vi "PH_PPMA_PowerUnit.panel.vi"() -> ()   [LabVIEW 2014, in "PH_PPMA_PowerUnit.lvlib"]
uses:
  PH_PPMA_PowerUnit.lvlib
  PH_PowerUnit_BaseClass/PH_PowerUnit_BaseClass.SM States.ctl
  PH_StatusHandler/PH_StatusHandler.GUI element.ctl
  PH_PowerUnit_BaseClass/PH_PowerUnit_BaseClass.GUI Refs to pack.ctl
  PH_PowerUnit_BaseClass/PH_PowerUnit_BaseClass.GUI Refs.ctl
  CSCore/CSObj/CSObj.lvlib
  PH_Common/PH_Common.lvlib
  PH_PowerUnit_BaseClass/PH_PowerUnit_BaseClass.lvlib
  PH_Class/PH_Class.lvlib
  PH_StatusHandler/PH_StatusHandler.lvlib
panel:
  out "Seq SM State":string
  out "PSDB Status":u32(colorbox)=6618880 caption="PSDB"
  out "Timing":u32(colorbox)
  out "Status":T1 caption="Enabling State"
  out "Timeout SM":T2 caption="State PU"
  out "State SM":T2 caption="State PU"
  out "Rods":u32(colorbox)
  out "Trigger":u32(colorbox)
  out "PSU":u32(colorbox)
  out "EOC":u32(colorbox)
  out "Ignitron":u32(colorbox)
  in  "PU on":bool
  out "Rossrelais":u32(colorbox) caption="Ross Relais"
  in  "Set Voltage":dbl
  in  "Exit":bool
  in  "Fire":bool
  out "Waiting Time":dbl
  out "Water Conductivity":u32(colorbox) caption="Water"
  out "Mercury":u32(colorbox)
  out "error out":errorcluster
  in  "Delete":bool
  in  "error in (no error)":errorcluster
  in  "object ref":refnum<vi>
  out "MainAmp":u32(colorbox)
  # "PCS"
  # "3.40"
  # "V"
  # "s"
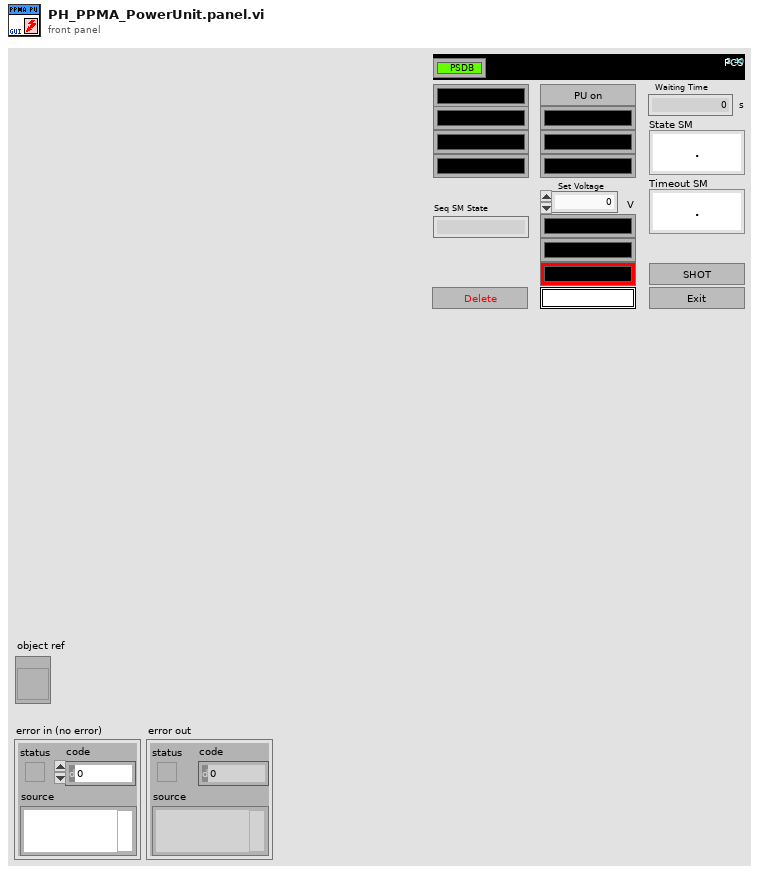
[diagram p1: front panel]
types:
  T1 = typedef "PH_StatusHandler.lvlib/PH_StatusHandler.GUI element.ctl" = u16
  T2 = typedef "PH_PowerUnit_BaseClass.lvlib/PH_PowerUnit_BaseClass.SM States.ctl" = enum16{".", "Stand by", "Switch PU on", "Configure", "Set Default Voltage", "Set STANDBY", "Set READY", "Wait for Shot Cmd", "Open Dump Rods", "Open Ross Relais", "Close Ross Relais", "Switch PSU on", "Switch PSU off", "Charge", "Switch GD Channel on", "Close Dump Rods", "Rods-TO", "RR-TO", "PSU-TO", "Trigger-TO"}
  T3 = typedef "PH_PowerUnit_BaseClass.lvlib/PH_PowerUnit_BaseClass.GUI Refs to pack.ctl" = cluster{"GUI Refs":T4, "Enabled":refnum<vi>, "PU on":refnum<vi>, "Waiting Time":refnum<vi>, "Timing.Instance":refnum<vi>, "Seq SM State":refnum<vi>, "Subscribed Trendmssgs":refnum<vi>[]}
  T4 = typedef "PH_PowerUnit_BaseClass.lvlib/PH_PowerUnit_BaseClass.GUI Refs.ctl" = cluster{"Delete Inst":refnum<vi>, "State TO SM":refnum<vi>, "State SM":refnum<vi>, "Fire":refnum<vi>}
  T5 = cluster{"GUI Refs Power Unit Base Class":T3, "PSDB Status":refnum<vi>}
  T6 = typedef "PH_PowerUnit_BaseClass.lvlib/PH_PowerUnit_BaseClass.i attribute.ctl" = cluster{"Constructor finished":bool, "PU":cluster{"In use":bool, "Service ID in use":i32, "GUI Ref":refnum<vi>}, "Enabling":cluster{"State":T7, "GUI Ref":refnum<vi>}, "Timing":cluster{"Last Shot":dbl, "Time between Shots [Sec]":dbl, "Waiting Time over?":bool, "Service ID Waiting Time":i32, "GUI Ref":refnum<vi>, "Instance":cluster{"Status":T8, "linked?":bool, "GUI Ref":refnum<vi>}}, "Sequencer":cluster{"SM State":string, "GUI Ref":refnum<vi>, "linked":bool}, "Subscribed Trendmssgs":cluster{"Tagname":string, "Status":T8, "linked?":bool, "Shot Condition":T8, "GUI Ref":refnum<vi>}[], "PP PU":T9, "Default Voltage (V)":dbl, "GUI Refs":T4, "PSDB data":cluster{"Shot Voltage [V]":dbl, "State TO SM":T2, "Write 2 early":bool}, "State TO SM":T2}
  T7 = typedef "PH_SystemInformation.lvlib/PH_SystemInformationEnabling State.ctl" = i32
  T8 = typedef "PH_StatusHandler.lvlib/PH_StatusHandler.Status.ctl" = i16
  T9 = typedef "PH_PP_Common.lvlib/PH_PP_Common.PUs.ctl" = enum16{"no Info", "PA-19mm-1", "PA-19mm-2", "PA-45mm-PILC", "PA-45mm-MAIN", "MA-PU-1", "MA-PU-2", "MA-PU-3", "MA-PU-4", "MA-PU-5", "MA-PU-6", "MA-FR", "MA-PILC", "PA-45mm-DP"}
  T10 = typedef "PH_PPMA_PowerUnit.lvlib/PH_PPMA_PowerUnit.i attribute.ctl" = cluster{"GUI Refs":cluster{"Rods":refnum<vi>, "Ignitron":refnum<vi>, "Rossrelais":refnum<vi>, "Set Voltage":refnum<vi>, "PSU":refnum<vi>, "EOC":refnum<vi>, "Trigger":refnum<vi>}, "Rods":T11, "PSU":T12, "Ross Relais":T13, "Ignitron":T14, "Trigger":cluster{"State Device":T8, "linked?":bool}, "Timing Settings":cluster{"Prdc Fast?":bool, "Default Value Periodic Interval":i32, "Mercury on since":dbl, "Warm up Time Mercury [s]":dbl}, "Set Voltage [V]":dbl}
  T11 = typedef "PH_PPMA_PowerUnit.lvlib/PH_PPMA_PowerUnit.Rods Attributes.ctl" = cluster{"Instancename":string, "Device Status":T8, "linked?":bool}
  T12 = typedef "PH_PP_Common.lvlib/PH_PP_Common.PSU Attributes.ctl" = cluster{"lower limit [V]":dbl, "upper limit [V]":dbl, "Voltage set":bool, "State Device":T8, "linked?":bool}
  T13 = typedef "PH_PP_Common.lvlib/PH_PP_Common.Ross Relais Attributes.ctl" = cluster{"State Device":T8, "linked?":bool}
  T14 = typedef "PH_PP_Common.lvlib/PH_PP_Common.Ignitron Attributes.ctl" = cluster{"State Device":T8, "linked?":bool}
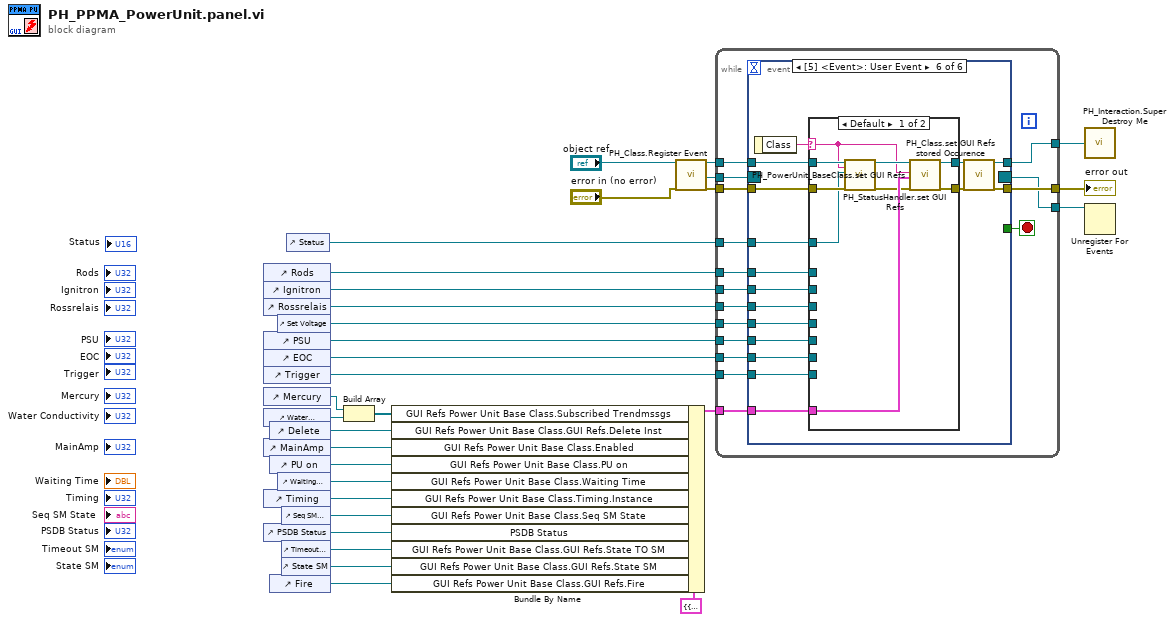
[diagram p0: block diagram]
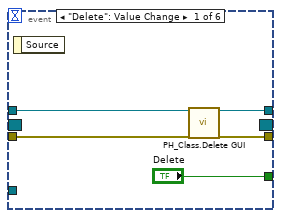
[diagram p2: hidden frame]
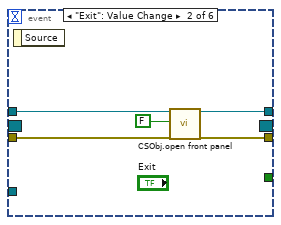
[diagram p3: hidden frame]
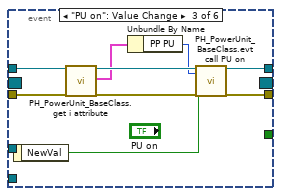
[diagram p4: hidden frame]
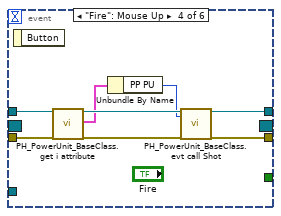
[diagram p5: hidden frame]
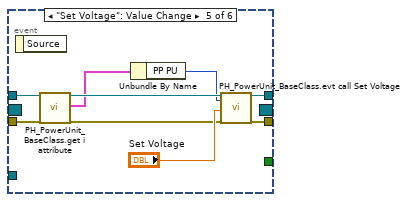
[diagram p6: hidden frame]
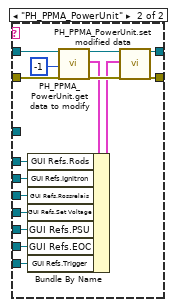
[diagram p7: hidden frame]
diagram:
  n1 = control-ref of="Rods"() -> (w22:refnum<vi>)
  n2 = control-ref of="Ignitron"() -> (w21:refnum<vi>)
  n3 = control-ref of="Rossrelais"() -> (w20:refnum<vi>)
  n4 = control-ref of="PSU"() -> (w18:refnum<vi>)
  n5 = control-ref of="EOC"() -> (w17:refnum<vi>)
  n6 = control-ref of="Trigger"() -> (w16:refnum<vi>)
  n7 = control-ref of="Mercury"() -> (w29:refnum<vi>)
  n8 = control-ref of="Water Conductivity"() -> (w27:refnum<vi>)
  n9 = control-ref of="MainAmp"() -> (w14:refnum<vi>)
  n10 = control-ref of="Timing"() -> (w11:refnum<vi>)
  n11 = control-ref of="PSDB Status"() -> (w8:refnum<vi>)
  n12 = control-ref of="Delete"() -> (w28:refnum<vi>)
  n13 = control-ref of="PU on"() -> (w13:refnum<vi>)
  n14 = control-ref of="Fire"() -> (w2:refnum<vi>)
  n15 = control-ref of="Set Voltage"() -> (w19:refnum<vi>)
  n16 = control-ref of="Waiting Time"() -> (w12:refnum<vi>)
  n17 = control-ref of="Seq SM State"() -> (w10:refnum<vi>)
  n18 = control-ref of="Timeout SM"() -> (w4:refnum<vi>)
  n19 = control-ref of="State SM"() -> (w3:refnum<vi>)
  n20 = control-ref of="Status"() -> (w1:refnum<vi>)
  n21 = Build Array(w29, w27) -> (w9:refnum<vi>[])
  n22 = Bundle By Name(cluster=T5 {"GUI Refs Power Unit Base Class"={"GUI Refs"={"Delete Inst"=refnum, "State TO SM"=refnum, "State SM"=refnum, "Fire"=refnum}, "Enabled"=refnum, "PU on"=refnum, "Waiting Time"=refnum, "Timing.Instance"=refnum, "Seq SM State"=refnum, "Subscribed Trendmssgs"=[]}, "PSDB Status"=refnum} ("GUI Refs"), "GUI Refs Power Unit Base Class.Subscribed Trendmssgs"=w9, "GUI Refs Power Unit Base Class.GUI Refs.Delete Inst"=w28, "GUI Refs Power Unit Base Class.Enabled"=w14, "GUI Refs Power Unit Base Class.PU on"=w13, "GUI Refs Power Unit Base Class.Waiting Time"=w12, "GUI Refs Power Unit Base Class.Timing.Instance"=w11, "GUI Refs Power Unit Base Class.Seq SM State"=w10, "PSDB Status"=w8, "GUI Refs Power Unit Base Class.GUI Refs.State TO SM"=w4, "GUI Refs Power Unit Base Class.GUI Refs.State SM"=w3, "GUI Refs Power Unit Base Class.GUI Refs.Fire"=w2) -> (w5:T5)
  n23 = call "PH_Class.Register Event.vi"("i ref in"="object ref", "error in (no error)"="error in (no error)") -> ("i ref out"=w26:refnum<vi>, "Event Registration Refnum"=w24:refnum<event-registration>, "error out"=w25:errorcluster)  [unwired: 15 in]
  n24 = while {
    tunnel: w26 -> [w44]
    tunnel: [w43] -> w31
    tunnel: [w46] -> w30
    tunnel: w25 -> [w45]
    tunnel: w24 -> [w42]
    tunnel: [w41] -> w23
    tunnel: w22 -> [w40]
    tunnel: w21 -> [w39]
    tunnel: w20 -> [w38]
    tunnel: w19 -> [w37]
    tunnel: w18 -> [w36]
    tunnel: w17 -> [w35]
    tunnel: w16 -> [w34]
    tunnel: w5 -> [w33]
    tunnel: w1 -> [w32]
    stop <- w47 stop-if-true
    n25 = event shown="[5] <Event>: User Event" {
      selector: w42 -> [_ _ _ _ _ _]
      dyn-events: [_ _ _ _ _ _] -> w41
      timeout: _ -> [_ _ _ _ _ _]
      tunnel: ["Delete" _ _ _ _ _] -> w47
      tunnel: w44 -> [w48 w55 w61 w70 w78 w99]
      tunnel: [w50 w56 w65 w73 w82 w94] -> w46
      tunnel: w45 -> [w51 w57 w66 w74 w83 w98]
      tunnel: [w49 w53 w63 w72 w80 w95] -> w43
      tunnel: w40 -> [_ _ _ _ _ w92]
      tunnel: w39 -> [_ _ _ _ _ w91]
      tunnel: w38 -> [_ _ _ _ _ w90]
      tunnel: w37 -> [_ _ _ _ _ w89]
      tunnel: w36 -> [_ _ _ _ _ w88]
      tunnel: w35 -> [_ _ _ _ _ w87]
      tunnel: w34 -> [_ _ _ _ _ w86]
      tunnel: w33 -> [_ _ _ _ _ w85]
      tunnel: w32 -> [_ _ _ _ _ w84]
      event "Delete": Value Change {
        n26 = event-data() -> ()  [unwired: 1 in, 1 out]
        n27 = call "PH_Class.Delete GUI.vi"("VI in"=w48, "error in (no error)"=w51) -> ("VI out"=w49:refnum<vi>, "error out"=w50:errorcluster)  [unwired: 16 in]
      }
      event "Exit": Value Change {
        n28 = event-data() -> ()  [unwired: 1 in, 1 out]
        n29 = call "CSObj.open front panel.vi"("i ref in"=w55, "frontPanelOpen"=FALSE ("front panel open"), "error in (no error)"=w57) -> ("i ref out"=w53:refnum<vi>, "error out"=w56:errorcluster)  [unwired: 15 in]
      }
      event "PU on": Value Change {
        n30 = event-data() -> ("NewVal"=w64:bool)  [unwired: 1 in]
        n31 = call "PH_PowerUnit_BaseClass.get i attribute.vi"("i ref in"=w61, "error in (no error)"=w66) -> ("i ref out"=w60:refnum<vi>, "i attribute"=w59:T6, "error out"=w62:errorcluster)  [unwired: 15 in]
        n32 = Unbundle By Name(w59) -> ("PP PU"=w58:T9)
        n33 = call "PH_PowerUnit_BaseClass.evt call PU on.vi"("i ref in"=w60, "PowerUnit"=w58, "PU on"=w64, "error in (no error)"=w62) -> ("i ref out"=w63:refnum<vi>, "error out"=w65:errorcluster)  [unwired: 14 in]
      }
      event "Fire": Mouse Up {
        n34 = event-data() -> ()  [unwired: 1 in, 1 out]
        n35 = call "PH_PowerUnit_BaseClass.get i attribute.vi"("i ref in"=w70, "error in (no error)"=w74) -> ("i ref out"=w69:refnum<vi>, "i attribute"=w68:T6, "error out"=w71:errorcluster)  [unwired: 15 in]
        n36 = Unbundle By Name(w68) -> ("PP PU"=w67:T9)
        n37 = call "PH_PowerUnit_BaseClass.evt call Shot.vi"("i ref in"=w69, "PowerUnit"=w67, "error in (no error)"=w71) -> ("i ref out"=w72:refnum<vi>, "error out"=w73:errorcluster)  [unwired: 15 in]
      }
      event "Set Voltage": Value Change {
        n38 = event-data() -> ()  [unwired: 1 in, 1 out]
        n39 = call "PH_PowerUnit_BaseClass.get i attribute.vi"("i ref in"=w78, "error in (no error)"=w83) -> ("i ref out"=w77:refnum<vi>, "i attribute"=w76:T6, "error out"=w79:errorcluster)  [unwired: 15 in]
        n40 = Unbundle By Name(w76) -> ("PP PU"=w75:T9)
        n41 = call "PH_PowerUnit_BaseClass.evt call Set Voltage.vi"("i ref in"=w77, "PowerUnit"=w75, "Voltage [V]"="Set Voltage", "error in (no error)"=w79) -> ("i ref out"=w80:refnum<vi>, "error out"=w82:errorcluster)  [unwired: 14 in]
      }
      event User Event {
        n42 = event-data() -> ("Class"=w93:string)  [unwired: 1 in]
        n43 = case shown="Default" w93 {
          selector: w93 -> [w101 _]
          tunnel: w99 -> [w103 w119]
          tunnel: w98 -> [w108 w118]
          tunnel: [w107 w117] -> w97
          tunnel: [w106 w116] -> w96
          tunnel: w92 -> [_ w115]
          tunnel: w91 -> [_ w114]
          tunnel: w90 -> [_ w113]
          tunnel: w89 -> [_ w112]
          tunnel: w88 -> [_ w111]
          tunnel: w87 -> [_ w110]
          tunnel: w86 -> [_ w109]
          tunnel: w85 -> [w105 _]
          tunnel: w84 -> [w100 _]
          frame Default {
            n44 = call "PH_StatusHandler.set GUI Refs.vi"("i ref in"=w103, "Class"=w101, "GUI Ref"=w100, "error in (no error)"=w108) -> ("i ref out"=w102:refnum<vi>, "error out"=w104:errorcluster)  [unwired: 14 in]
            n45 = call "PH_PowerUnit_BaseClass.set GUI Refs.vi"("i ref  in"=w102, "Class"=w101, "GUI Refs"=w105, "error in"=w104) -> ("i ref out"=w107:refnum<vi>, "error out"=w106:errorcluster)  [unwired: 14 in]
          }
          frame "PH_PPMA_PowerUnit" {
            n46 = call "PH_PPMA_PowerUnit.get data to modify.vi"("i ref in"=w119, "ms timeout (10000)"=-1, "error in (no error)"=w118) -> ("i ref out"=w122:refnum<vi>, "i attribute"=w121:T10, "error out"=w124:errorcluster)  [unwired: 13 in, 1 out]
            n47 = Bundle By Name(cluster=w121, "GUI Refs.Rods"=w115, "GUI Refs.Ignitron"=w114, "GUI Refs.Rossrelais"=w113, "GUI Refs.Set Voltage"=w112, "GUI Refs.PSU"=w111, "GUI Refs.EOC"=w110, "GUI Refs.Trigger"=w109) -> (w120:T10)
            n48 = call "PH_PPMA_PowerUnit.set modified data.vi"("i ref in"=w122, "i attribute"=w120, "error in (no error)"=w124) -> ("i ref out"=w117:refnum<vi>, "error out"=w116:errorcluster)  [unwired: 15 in]
          }
        }
        n49 = call "PH_Class.set GUI Refs stored Occurence.vi"("i ref in"=w97, "error in (no error)"=w96) -> ("i ref out"=w95:refnum<vi>, "error out"=w94:errorcluster)  [unwired: 16 in]
      }
    }
  }
  "error out" <- w30
  n50 = call "PH_Interaction.Super Destroy Me.vi"("i ref out"=w31) -> ()
  n51 = Unregister For Events(event registration refnum=w23) -> ()  [unwired: 1 in, 1 out]
